vi "Set Output Enable.vi"(8 "error in (no error)":errorcluster, 10 "Enabled?":bool, 11 "LINX-SN3218 in":refnum<class "LINX-SN3218.lvclass">) -> (0 "error out":errorcluster, 3 "LINX-SN3218 out":refnum<class "LINX-SN3218.lvclass">)   [LabVIEW 2020, in "LINX-SN3218.lvclass"]
uses:
  LINX-SN3218.lvclass
  LINX I2C/LINX I2C.lvclass
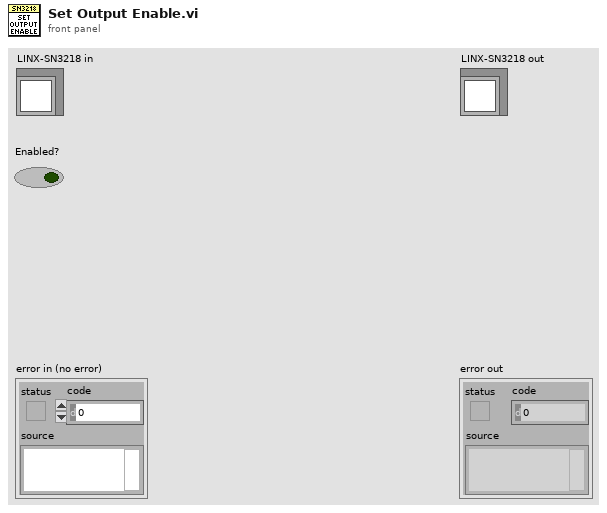
[diagram p1: front panel]
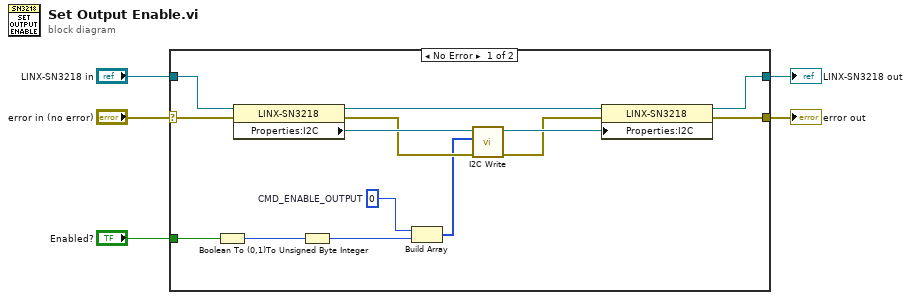
[diagram p0: block diagram]
diagram:
  n1 = case shown="No Error" "error in (no error)" {
    selector: "error in (no error)" -> [w17 w21]
    tunnel: [w11 w21] -> w4
    tunnel: [w15 w20] -> w2
    tunnel: "LINX-SN3218 in" -> [w19 w20]
    tunnel: "Enabled?" -> [w10 _]
    frame No Error {
      w7 = u8 0  # CMD_ENABLE_OUTPUT
      n2 = Boolean To (0,1)(Boolean=w10) -> (0, 1=w9:i16)
      n3 = property class="LINX-SN3218"(reference=w19, error in=w17) -> (reference out=w16:refnum<class "LINX-SN3218.lvclass">, error out=w13:errorcluster, "Properties:I2C"=w18:refnum<class "LINX I2C.lvclass">)
      n4 = To Unsigned Byte Integer(number=w9) -> (unsigned 8bit integer=w8:u8)
      n5 = Build Array(w7, w8) -> (w6:u8[])
      n6 = call "I2C Write.vi"("error in (no error)"=w13, "Bytes to Write"=w6, "LINX I2C in"=w18) -> ("error out"=w12:errorcluster, "LINX I2C out"=w14:refnum<class "LINX I2C.lvclass">)  [unwired: 7 in]
      n7 = property class="LINX-SN3218"(reference=w16, error in=w12, "Properties:I2C"=w14) -> (reference out=w15:refnum<class "LINX-SN3218.lvclass">, error out=w11:errorcluster)
    }
    frame Error {
    }
  }
  "error out" <- w4
  "LINX-SN3218 out" <- w2
